vi "_RT_CtrlLoop_Laser_WriteSetting.vi"(8 "error in (no error)":errorcluster, 10 "input cluster":T1={"Energy"=50.0, "Freq"=100.0, "Emission"=FALSE, "TriggerSource"=enum."Internal", "Time Stamp"=timestamp(0 s since 1904-01-01)}, 11 "Laser349 in":refnum<class "Laser349.lvclass">) -> (0 "error out":errorcluster, 3 "Laser349 out":refnum<class "Laser349.lvclass">)   [LabVIEW 2018]
uses:
  Ctl/_ctl_LaserParam.ctl
  Class/Laser349.lvclass
  Ctl/_ctl_LaserCmd.ctl
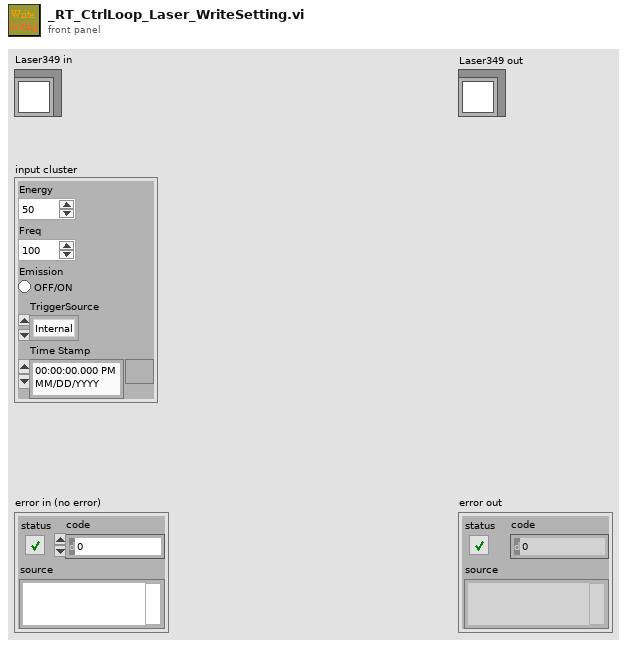
[diagram p1: front panel]
types:
  T1 = typedef "_ctl_LaserParam.ctl" = cluster{"Energy":dbl, "Freq":dbl, "Emission":bool, "TriggerSource":enum16{"Internal", "External"}, "Time Stamp":timestamp}
  T2 = typedef "_ctl_LaserCmd.ctl" = enum8{"Diode_On", "Diode_Off", "Standby_On", "Standby_Off", "Internal_Trig", "External_Trig", "Set_Energy", "Set_Frequency", "Read_Version", "Read_STB", "Read_Diode_TEMP", "Read_SHG_TEMP", "Read_THG_TEMP", "Read_Base_Plate_TEMP", "Read_Diode_Hour", "Read_Diode_Maxc", "Read_Diode_Curr", "Read_QSW_CNTS", "Read_PENER", "Read_Freq", "Read_PCUR", "Read_Fault_Codes"}
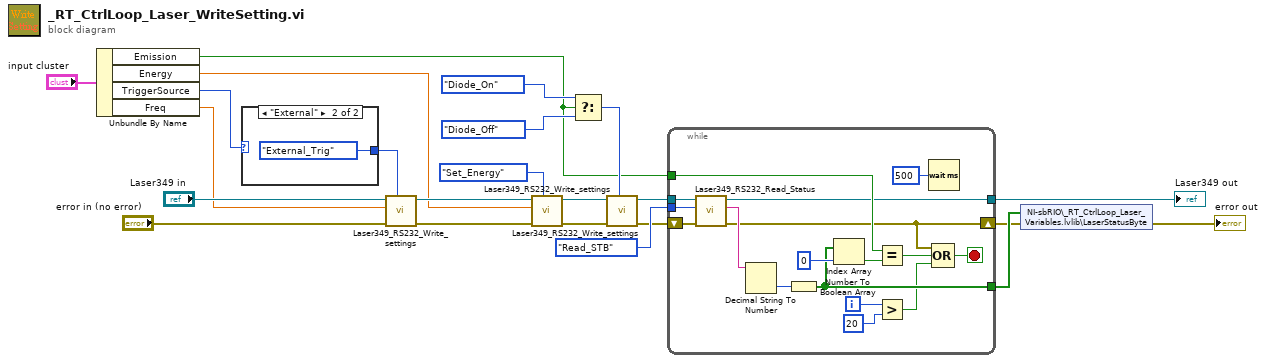
[diagram p0: block diagram]
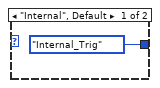
[diagram p2: hidden frame]
diagram:
  n1 = Unbundle By Name("input cluster") -> ("Emission"=w7:bool, "Energy"=w2:dbl, "TriggerSource"=w10:enum16{"Internal", "External"}, "Freq"=w11:dbl)
  n2 = case shown="\"External\"" w10 {
    tunnel: [_ctl_LaserCmd."Internal_Trig" ("Command Status") _ctl_LaserCmd."External_Trig" ("Command Status")] -> w15
    frame "Internal", Default {
    }
    frame "External" {
    }
  }
  n3 = call-dynamic "Laser349_RS232_Write_settings.vi"("Command Status"=w15, "error in (no error)"="error in (no error)", "Input value"=w11, "Laser349 in"="Laser349 in") -> ("error out"=w9:errorcluster, "Laser349 out"=w19:refnum<class "Laser349.lvclass">)  [unwired: 6 in]
  n4 = call-dynamic "Laser349_RS232_Write_settings.vi"("Command Status"=_ctl_LaserCmd."Set_Energy", "error in (no error)"=w9, "Input value"=w2, "Laser349 in"=w19) -> ("error out"=w16:errorcluster, "Laser349 out"=w17:refnum<class "Laser349.lvclass">)  [unwired: 6 in]
  n5 = Select(t=_ctl_LaserCmd."Diode_On" ("Command Status"), s=w7, f=_ctl_LaserCmd."Diode_Off" ("Command Status")) -> (s? t:f=w18:T2)
  n6 = call-dynamic "Laser349_RS232_Write_settings.vi"("Command Status"=w18, "error in (no error)"=w16, "Laser349 in"=w17) -> ("error out"=w6:errorcluster, "Laser349 out"=w4:refnum<class "Laser349.lvclass">)  [unwired: 7 in]
  n7 = while {
    tunnel: _ctl_LaserCmd."Read_STB" ("Command Status") -> [w40]
    shift-right: [w31] -> w3
    shift-left: w6 -> [w39]
    tunnel: w7 -> [w36]
    tunnel: [w35] -> w5
    tunnel: w4 -> [w33]
    tunnel: [w32] -> w23
    i -> [w28]
    stop <- w29 stop-if-true
    n8 = call-dynamic "Laser349_RS232_Read_Status.vi"("error in (no error)"=w39, "Command Status"=w40, "Laser349 in"=w33) -> ("error out"=w31:errorcluster, "Result String"=w41:string, "Laser349 out"=w32:refnum<class "Laser349.lvclass">)  [unwired: 6 in]
    n9 = Decimal String To Number(string=w41) -> (number=w42:i32)  [unwired: 2 in, 1 out]
    n10 = Number To Boolean Array(number=w42) -> (Boolean array=w35:bool[])
    n11 = Index Array(array=w35, index=0) -> (element=w34:bool)
    n12 = Equal?(x=w36, y=w34) -> (x = y?=w30:bool)
    n13 = Greater?(x=w28, y=20) -> (0:w26:bool)
    n14 = Wait (ms)(milliseconds to wait=u32 500) -> ()  [unwired: 1 out]
    n15 = Compound Arithmetic op=OR(w31, w30, w26) -> (w29:bool)
  }
  "Laser349 out" <- w23
  n16 = shared-variable "NI-sbRIO\\_RT_CtrlLoop_Laser_Variables.lvlib\\LaserStatusByte"(w5, error in=w3) -> (error out=→"error out":errorcluster)
